vi "Handle Token Response.vi"(8 "error in (no error)":errorcluster, 10 "Response Body":string, 11 "Async Authorization in":refnum<class "Async Authorization.lvclass">) -> (0 "error out":errorcluster, 3 "Asyn Authorization out":refnum<class "Async Authorization.lvclass">)   [LabVIEW 2020, in "OAuth2.lvlib" / "Async Authorization.lvclass"]
uses:
  Async Authorization.lvclass
  Async Authorization.lvclass/Async Authorization.ctl
  Authorization/Authorization.lvclass
  <vilib>/IlluminatedG/lv-web-crypto/lv-json/JSON/JSON.lvlib
  <vilib>/JDP Science/JSONtext/JSONtext.lvlib
  3b40fd08-d5a5-4162-adab-a042d9031a6d.vi
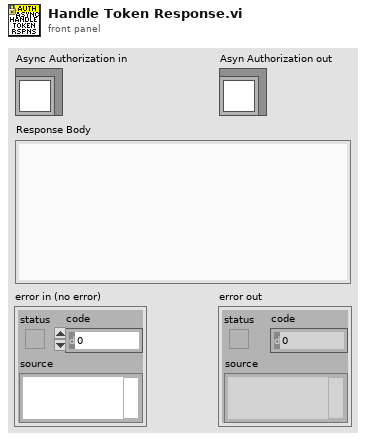
[diagram p1: front panel]
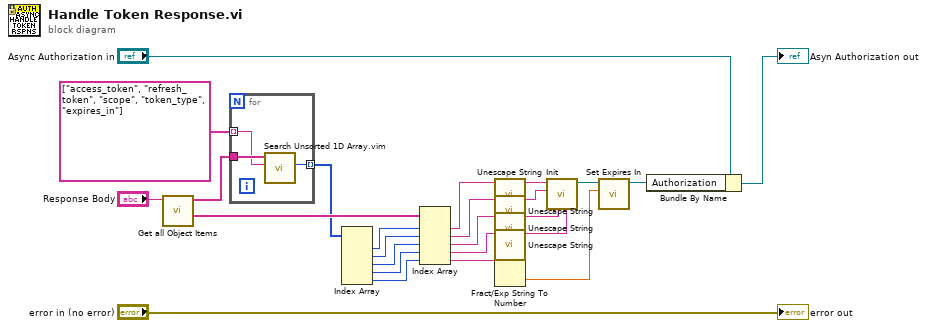
[diagram p0: block diagram]
diagram:
  n1 = call <vilib>:"Get all Object Items.vi"("JSON"="Response Body") -> ("<JSON>"=w8:string[], "Item Names"=w9:string[])  [unwired: 7 in, 2 out]
  n2 = for {
    tunnel: w9 -> [w28]
    tunnel: string[] ["access_token", "refresh_token", "scope", "token_type", "expires_in"] ("Search Keys") -> [w27] mode=indexing
    tunnel: [w26] -> w6 mode=indexing
    n3 = call "Search Unsorted 1D Array.vim"("element"=w27, "unsorted 1D array"=w28) -> ("index of element"=w26:i32)  [unwired: 9 in]
  }
  n4 = Index Array(array=w6) -> (element #1=w5:i32, element #2=w4:i32, element #3=w3:i32, element #4=w2:i32, element #5=w1:i32)  [unwired: 5 in]
  n5 = Index Array(array=w8, index #1=w5, index #2=w4, index #3=w3, index #4=w2, index #5=w1) -> (element #1=w18:string, element #2=w15:string, element #3=w14:string, element #4=w12:string, element #5=w24:string)
  n6 = call <vilib>:"Unescape String.vi"("Escaped String"=w18) -> ("String"=w17:string)  [unwired: 10 in]
  n7 = call <vilib>:"Unescape String.vi"("Escaped String"=w15) -> ("String"=w16:string)  [unwired: 10 in]
  n8 = call <vilib>:"Unescape String.vi"("Escaped String"=w14) -> ("String"=w13:string)  [unwired: 10 in]
  n9 = call <vilib>:"Unescape String.vi"("Escaped String"=w12) -> ("String"=w11:string)  [unwired: 10 in]
  n10 = Fract/Exp String To Number(string=w24) -> (number=w22:dbl)  [unwired: 3 in, 1 out]
  n11 = call "Init.vi"("Token Type"=w11, "Scope"=w13, "Refresh Token"=w16, "Access Token"=w17) -> ("Authorization"=w23:refnum<class "Authorization.lvclass">)  [unwired: 7 in]
  n12 = call "Set Expires In.vi"("Expires In"=w22, "Authorization in"=w23) -> ("Authorization out"=w21:refnum<class "Authorization.lvclass">)  [unwired: 9 in]
  n13 = Bundle By Name(cluster="Async Authorization in", "Authorization"=w21) -> (→"Asyn Authorization out":refnum<class "Async Authorization.lvclass">)
  "error out" <- "error in (no error)"
